vi "ReadUDP.vi"(2 "error in (no error)":errorcluster, 3 "connection ID":refnum<k16>, 4 "Message length":u16=10) -> (0 "error out":errorcluster, 1 "Array":u8[][](array[numeric])=[[2, 225, 14, 196, 12, 0, 0, 0, 0, 0], [2, 226, 35, 253, 12, 0, 0, 0, 0, 0], [2, 227, 56, 248, 12, 0, 0, 0, 0, 0], [2, 228, 77, 195, 12, 0, 0, 0, 0, 0], [2, 241, 7, 28, 0, 0, 0, 0, 0, 0], [2, 242, 14, 27, 0, 0, 0, 0, 0, 0], [2, 243, 21, 29, 0, 0, 0, 0, 0, 0], [2, 244, 28, 28, 0, 0, 0, 0, 0, 0], [0, 144, 12, 42, 12, 247, 12, 20, 12, 129], [0, 112, 11, 37, 0, 225, 1, 0, 0, 0], [0, 113, 15, 104, 8, 4, 1, 0, 0, 0], [2, 0, 2, 4, 5, 5, 2, 0, 0, 0], [0, 98, 3, 242, 1, 24, 0, 131, 0, 0], [0, 99, 46, 33, 1, 1, 1, 1, 1, 44], [0, 102, 2, 71, 1, 51, 0, 74, 0, 0], [0, 103, 33, 35, 1, 1, 1, 1, 1, 44]])   [LabVIEW 2017]
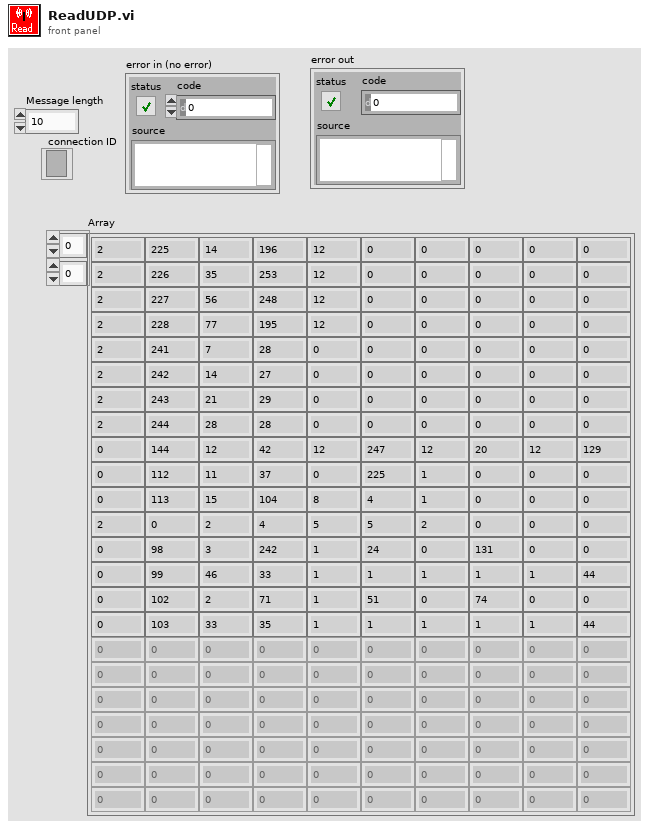
[diagram p1: front panel]
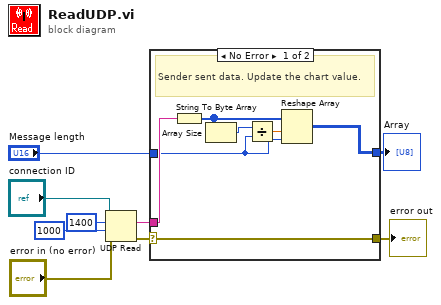
[diagram p0: block diagram]
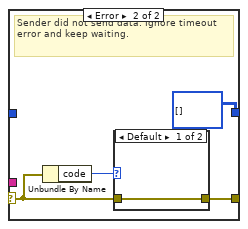
[diagram p2: hidden frame]
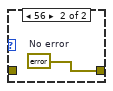
[diagram p3: hidden frame]
diagram:
  n1 = UDP Read(connection ID="connection ID", max size (548)=1400, timeout ms (25000)=1000, 8:"error in (no error)") -> (data out=w6:string, error out=w7:errorcluster)  [unwired: 3 out]
  n2 = case shown="No Error" w7 {
    selector: w7 -> [w16 w19]
    tunnel: w6 -> [w15 _]
    tunnel: [w16 w18] -> w1
    tunnel: [w11 u8[][] [] ("unsigned byte array")] -> w5
    tunnel: "Message length" -> [w10 _]
    frame No Error {
      # "Sender sent data. Update the chart value."
      n3 = String To Byte Array(string=w15) -> (unsigned byte array=w14:u8[])
      n4 = Array Size(array=w14) -> (size(s)=w13:i32)
      n5 = Divide(x=w13, y=w10) -> (x/y=w12:dbl)
      n6 = Reshape Array(w14, w12, w10) -> (w11:u8[][])
    }
    frame Error {
      # "Sender did not send data. Ignore timeout error and keep waiting."
      n7 = Unbundle By Name(w19) -> ("code"=w20:i32)
      n8 = case shown="Default" w20 {
        tunnel: w19 -> [w21 _]
        tunnel: [w21 w22] -> w18
        frame Default {
        }
        frame 56 {
          w22 = errorcluster {"status"=FALSE, "code"=0, "source"=""}  # No error
        }
      }
    }
  }
  "Array" <- w5
  "error out" <- w1
